vi "Online Detrend and Trend Estimation.vi"() -> ()   [LabVIEW 2023]
doc: "This example shows how to remove trends from a streaming signal using the WA Online Detrend VI.\n\n<b>Instructions:</b>\n1) Run this VI.\n2) Change the <b>Wavelet</b> type and <b>Threshold frequency</b>.\n3) Observe the detrending performance in the <b>Signal and Trend Signal</b> and <b>Detrended Signal</b> graphs."
uses:
  <vilib>/addons/Wavelet Analysis/online wavelet analysis.llb/WA Online Detrend (Array).vi
  <vilib>/addons/_Advanced Signal Processing/NI_AdvSigProcOnlineWA.lvlib
  <vilib>/Analysis/NI_AALBase.lvlib
panel:
  out "Detrended Signal":dbl[](graph)
  in  "stop":bool
  out "Signal and Trend Signal":dbl[][](graph)
  in  "Wavelet":u16(ring) items=["db02"=0, "db03"=1, "db04"=2, "db05"=3, "db06"=4, "db07"=5, "db08"=6, "db09"=7, "db10"=8, "db11"=9, "db12"=10, "db13"=11, "db14"=12, "Haar"=13, "bior1_3"=14, "bior1_5"=15, "bior2_2"=16, "bior2_4"=17, "bior2_6"=18, "bior2_8"=19, "bior3_1"=20, "bior3_3"=21, "bior3_5"=22, "bior3_7"=23, "bior3_9"=24, "bior4_4 (FBI)"=25, "bior5_5"=38, "bior6_8"=39, "coif1"=26, "coif2"=27, "coif3"=28, "coif4"=29, "coif5"=30, "sym2"=31, "sym3"=32, "sym4"=33, "sym5"=34, "sym6"=35, "sym7"=36, "sym8"=37]
  in  "Threshold frequency":dbl=0.031200000000000002 min=0.001 max=0.5 step=0.0001 format="%.4f"
  # "Overview: Shows how to remove trends from a streaming signal using the WA Online Detrend VI.\nRequirements: LabVIEW Full Development System, Advanced Signal Processing Toolkit\nInstructions: \n1. Run this VI.\n2. Change the Wavelet type and Threshold frequency.\n3. Observe the detrending performance in the Signal and Trend Signal and Detrended Signal graphs.\n4. Click Stop to stop the VI."
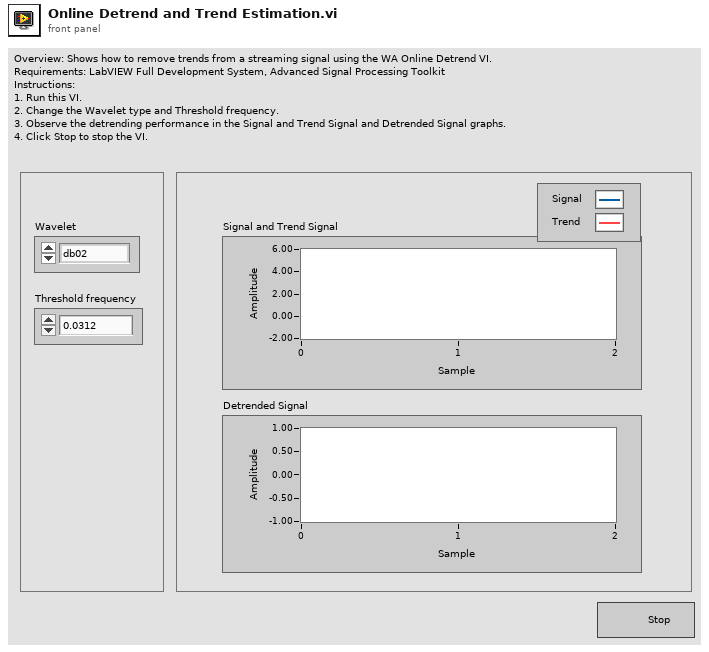
[diagram p1: front panel]
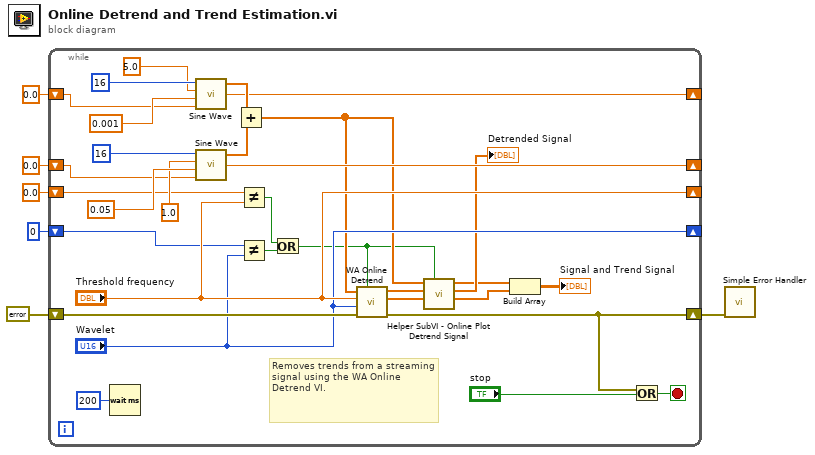
[diagram p0: block diagram]
diagram:
  n1 = while {
    shift-right: [w26] -> _
    shift-left: 0.0 ("phase out") -> [w24]
    shift-right: [w25] -> _
    shift-left: 0.0 ("phase out") -> [w23]
    shift-right: [w7] -> w1
    shift-left: errorcluster {"status"=FALSE, "code"=0, "source"=""} ("error out") -> [w22]
    shift-right: ["Threshold frequency"] -> _
    shift-left: 0.0 ("Threshold frequency") -> [w21]
    shift-right: ["Wavelet"] -> _
    shift-left: u16 0 ("Wavelet") -> [w19]
    stop <- w36 stop-if-true
    # "Removes trends from a streaming signal using the WA Online Detrend VI."
    n2 = Wait (ms)(milliseconds to wait=u32 200 ("millisecond multiple")) -> ()  [unwired: 1 out]
    n3 = call <vilib>:"Sine Wave.vi"("samples"=16, "amplitude"=5.0, "frequency"=0.001 ("phase(degrees)"), "phase in"=w24) -> ("sine wave"=w28:dbl[], "phase out"=w26:dbl)  [unwired: 1 in, 1 out]
    n4 = call <vilib>:"Sine Wave.vi"("samples"=16, "amplitude"=1.0, "frequency"=0.05 ("phase(degrees)"), "phase in"=w23) -> ("sine wave"=w27:dbl[], "phase out"=w25:dbl)  [unwired: 1 in, 1 out]
    n5 = Add(x=w28, y=w27) -> (x+y=w13:dbl[])
    n6 = Not Equal?(x=w21, y="Threshold frequency") -> (x != y?=w17:bool)
    n7 = Not Equal?(x=w19, y="Wavelet") -> (x != y?=w16:bool)
    n8 = Or(x=w17, y=w16) -> (x .or. y?=w11:bool)
    n9 = call-poly <vilib>:"WA Online Detrend.vi"("initialize? (F)"=w11, "error in (no error)"=w22, "wavelet"="Wavelet", "threshold frequency"="Threshold frequency", "signal"=w13) -> ("error out"=w7:errorcluster, "trend signal"=w15:dbl[], "detrended signal"=w14:dbl[])  [unwired: 4 in]
    n10 = call "Helper SubVI - Online Plot Detrend Signal.vi"("initialize? (F)"=w11, "trend signal"=w15, "detrended signal"=w14, "signal"=w13) -> ("trend signal out"=w9:dbl[], "detrended signal out"=→"Detrended Signal":dbl[], "signal out"=w10:dbl[])  [unwired: 5 in]
    n11 = Build Array(w10, w9) -> (→"Signal and Trend Signal":dbl[][])
    n12 = Or(x=w7, y="stop") -> (x .or. y?=w36:bool)
  }
  n13 = call <vilib>:"Simple Error Handler.vi"("error in (no error)"=w1) -> ()  [unwired: 1 in, 8 out]
